vi "RX-TX-BPCS-HMI-Modbus (SubVI).vi"(0 "Modbus Slave in":refnum<class "Modbus Slave.lvclass">, 1 "SIM-BPCS-RX-ARRAY":dbl[](array[numeric]), 3 "SIS-BPCS-RX-Array":bool[](array[boolean]), 4 "BPCS-SIM-TX-ARRAY":dbl[](array[numeric]), 5 "error in (no error)":errorcluster) -> (7 "HMI-10HIC300":dbl, 8 "HMI-10LIC200-KPID":dbl[](array[numeric]), 10 "HMI-10LIC200_MA":bool, 11 "HMI-10HIC100":dbl, 12 "HMI-10TIC100_MA":bool, 13 "HMI-10TIC100-KPID":dbl[](array[numeric]), 14 "Modbus Slave out":refnum<class "Modbus Slave.lvclass">, 15 "HMI-10LIC200-SP":dbl, 17 "HMI-10HIC200":dbl, 18 "HMI-10TIC100-SP":dbl, 19 "error out":errorcluster)   [LabVIEW 2018]
uses:
  <vilib>/Modbus/slave/Modbus Slave.lvclass
panel:
  out "BPCS-HMI-TX-ARRAY":dbl[](array[numeric])
  out "register values":u16[](array[numeric])
  in  "Array in":dbl[](array[numeric])
  in  "type 2":u16[](array[numeric])
  in  "type":u16[](array[numeric])
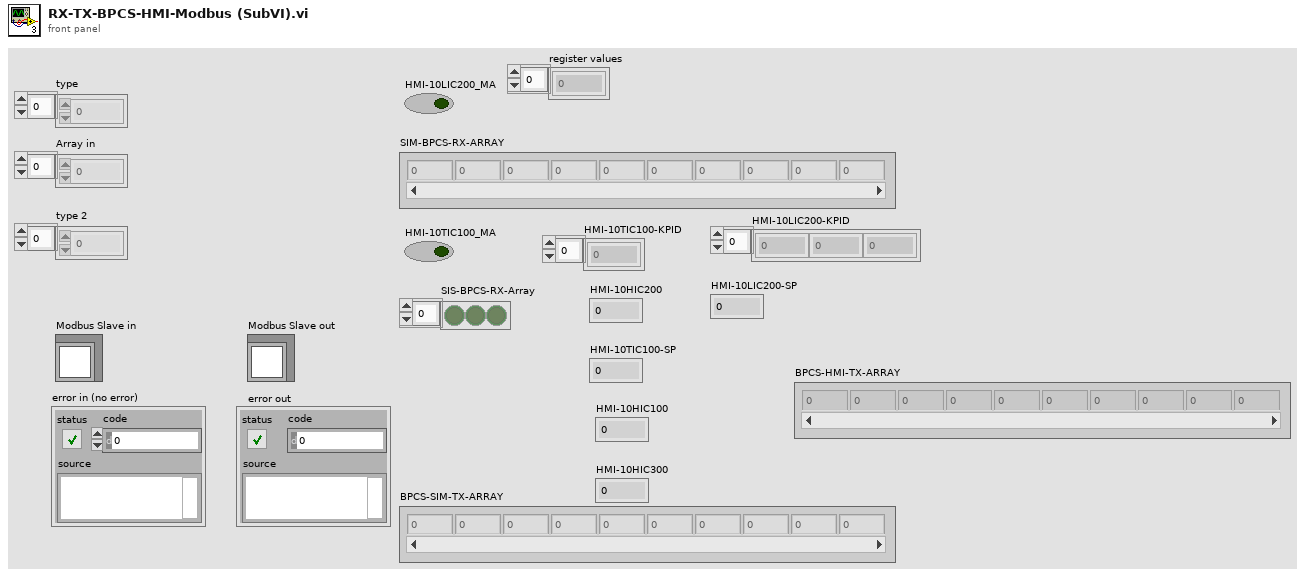
[diagram p1: front panel]
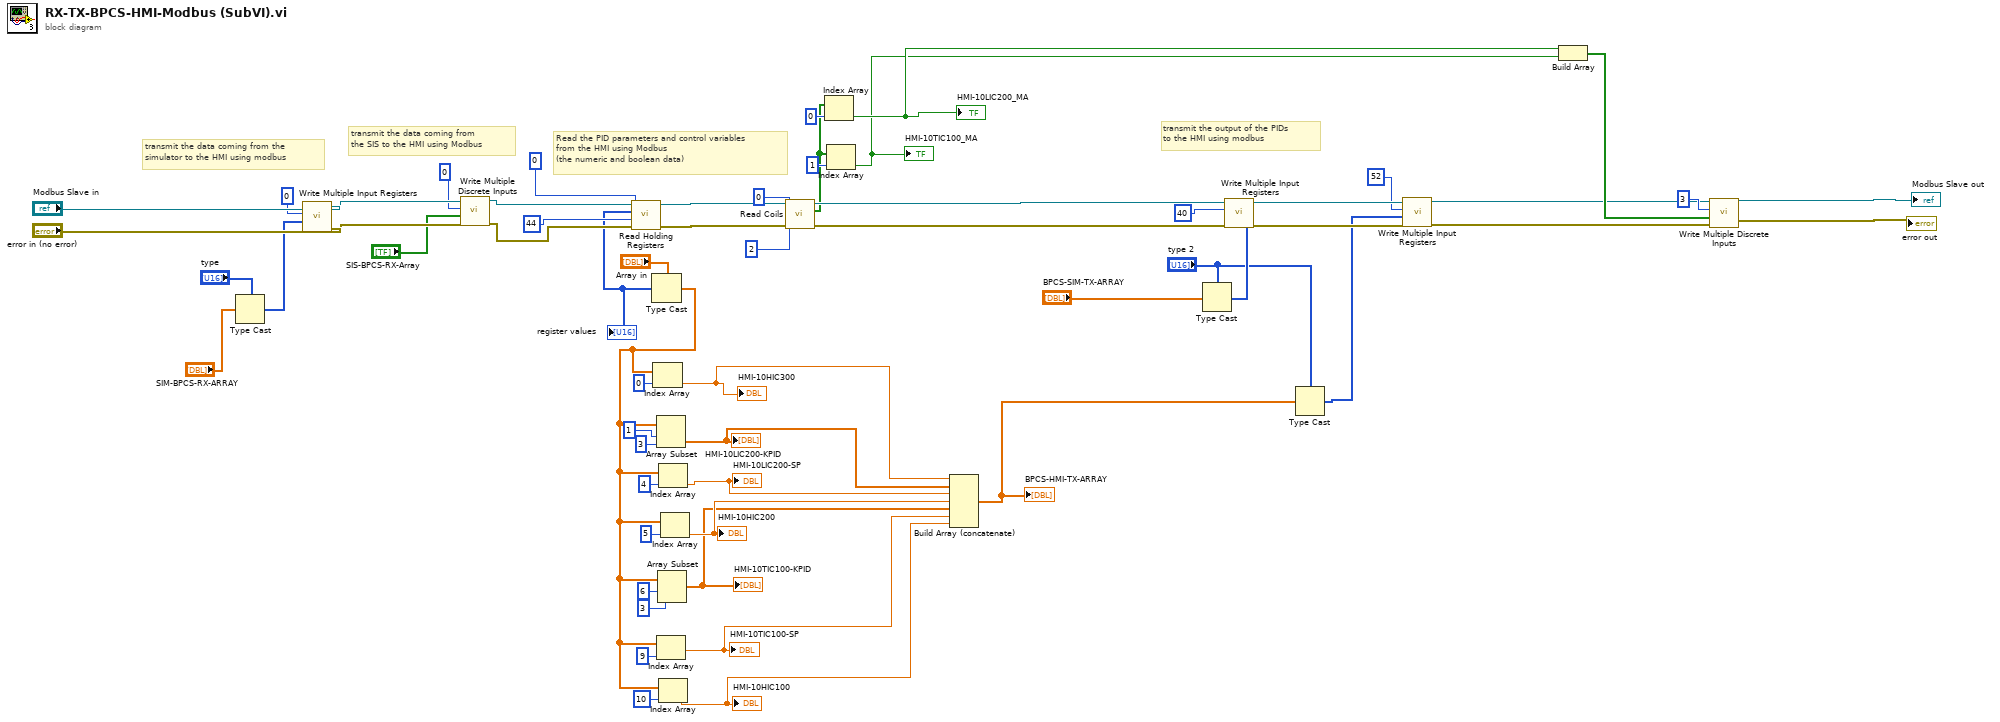
[diagram p0: block diagram]
diagram:
  # "transmit the output of the PIDs \nto the HMI using modbus"
  # "Read the PID parameters and control variables \nfrom the HMI using Modbus\n(the numeric and boolean data)"
  # "transmit the data coming from \nthe SIS to the HMI using Modbus"
  # "transmit the data coming from the \nsimulator to the HMI using modbus"
  n1 = Type Cast(type="type", x="SIM-BPCS-RX-ARRAY") -> (*(type *) &x=w51:u16[])
  n2 = call-dynamic "Write Multiple Input Registers.vi"("error in (no error)"="error in (no error)", "input register values"=w51, "starting address"=u16 0, "Modbus slave in"="Modbus Slave in") -> ("error out"=w57:errorcluster, "Modbus slave out"=w56:refnum<class "Modbus Slave.lvclass">)  [unwired: 6 in]
  n3 = call-dynamic "Write Multiple Discrete Inputs.vi"("error in (no error)"=w57, "discrete input values"="SIS-BPCS-RX-Array", "starting address"=u16 0, "Modbus slave in"=w56) -> ("error out"=w54:errorcluster, "Modbus slave out"=w55:refnum<class "Modbus Slave.lvclass">)  [unwired: 6 in]
  n4 = call-dynamic "Read Holding Registers.vi"("error in (no error)"=w54, "number of holding registers"=u16 44, "starting address"=u16 0, "Modbus slave in"=w55) -> ("error out"=w28:errorcluster, "register values"=w26:u16[], "Modbus slave out"=w29:refnum<class "Modbus Slave.lvclass">)  [unwired: 5 in]
  "register values" <- w26
  n5 = Type Cast(type="Array in", x=w26) -> (*(type *) &x=w9:dbl[])
  n6 = Index Array(array=w9, index=0) -> (element=w1:dbl)
  "HMI-10HIC300" <- w1
  n7 = Array Subset(array=w9, index=1, length=3) -> (w8:dbl[])
  "HMI-10LIC200-KPID" <- w8
  n8 = Index Array(array=w9, index=9) -> (element=w4:dbl)
  "HMI-10TIC100-SP" <- w4
  n9 = Array Subset(array=w9, index=6, length=3) -> (w5:dbl[])
  "HMI-10TIC100-KPID" <- w5
  n10 = Index Array(array=w9, index=4) -> (element=w7:dbl)
  "HMI-10LIC200-SP" <- w7
  n11 = Index Array(array=w9, index=10) -> (element=w3:dbl)
  "HMI-10HIC100" <- w3
  n12 = Index Array(array=w9, index=5) -> (element=w6:dbl)
  "HMI-10HIC200" <- w6
  n13 = call-dynamic "Read Coils.vi"("error in (no error)"=w28, "number of coils"=u16 2, "starting address"=u16 0, "Modbus slave in"=w29) -> ("error out"=w52:errorcluster, "coil values"=w27:bool[], "Modbus slave out"=w53:refnum<class "Modbus Slave.lvclass">)  [unwired: 5 in]
  n14 = Index Array(array=w27, index=0) -> (element=w20:bool)
  "HMI-10LIC200_MA" <- w20
  n15 = Index Array(array=w27, index=1) -> (element=w19:bool)
  "HMI-10TIC100_MA" <- w19
  n16 = Build Array (concatenate)(w1, w8, w7, w6, w5, w4, w3) -> (w2:dbl[])
  "BPCS-HMI-TX-ARRAY" <- w2
  n17 = Type Cast(type="type 2", x="BPCS-SIM-TX-ARRAY") -> (*(type *) &x=w24:u16[])
  n18 = call-dynamic "Write Multiple Input Registers.vi"("error in (no error)"=w52, "input register values"=w24, "starting address"=u16 40, "Modbus slave in"=w53) -> ("error out"=w15:errorcluster, "Modbus slave out"=w16:refnum<class "Modbus Slave.lvclass">)  [unwired: 6 in]
  n19 = Type Cast(type="type 2", x=w2) -> (*(type *) &x=w11:u16[])
  n20 = call-dynamic "Write Multiple Input Registers.vi"("error in (no error)"=w15, "input register values"=w11, "starting address"=u16 52, "Modbus slave in"=w16) -> ("error out"=w13:errorcluster, "Modbus slave out"=w14:refnum<class "Modbus Slave.lvclass">)  [unwired: 6 in]
  n21 = Build Array(w20, w19) -> (w18:bool[])
  n22 = call-dynamic "Write Multiple Discrete Inputs.vi"("error in (no error)"=w13, "discrete input values"=w18, "starting address"=u16 3, "Modbus slave in"=w14) -> ("error out"=→"error out":errorcluster, "Modbus slave out"=→"Modbus Slave out":refnum<class "Modbus Slave.lvclass">)  [unwired: 6 in]
